vi "tcpServer.vi"(8 "error in (no error)":errorcluster, 11 "TcpServer in":refnum<class "TcpServer.lvclass">) -> (0 "error out":errorcluster, 3 "TcpServer out":refnum<class "TcpServer.lvclass">)   [LabVIEW 2018, in "TcpServer.lvclass"]
doc: "This is the Tcp Server that receives packets from Python Client, send acknowledgement to client and manage the incommiing and outcomming events."
uses:
  TcpServer.lvclass
  TcpServer.lvclass/TcpServer.ctl
panel:
  out "Packet":string
  out "Client IP":string
  out "error tcp":errorcluster
  out "Packet In":string
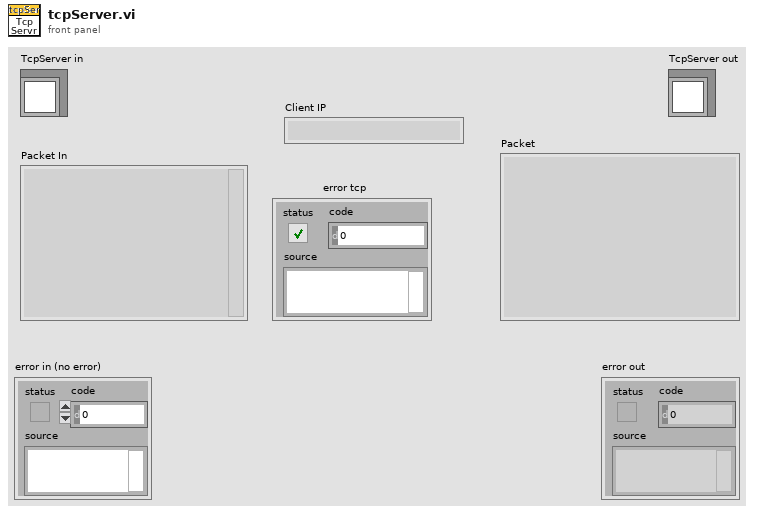
[diagram p1: front panel]
types:
  T1 = typedef "TcpServer.lvclass/userEventsTypeDef.ctl" = cluster{"TcpServer":refnum<user-event>, "Command":refnum<user-event>, "Ack":refnum<user-event>, "Event":refnum<user-event>, "Telemetry":refnum<user-event>}
  T2 = enum16{"Standard", "Buffered", "CRLF", "Immediate"}
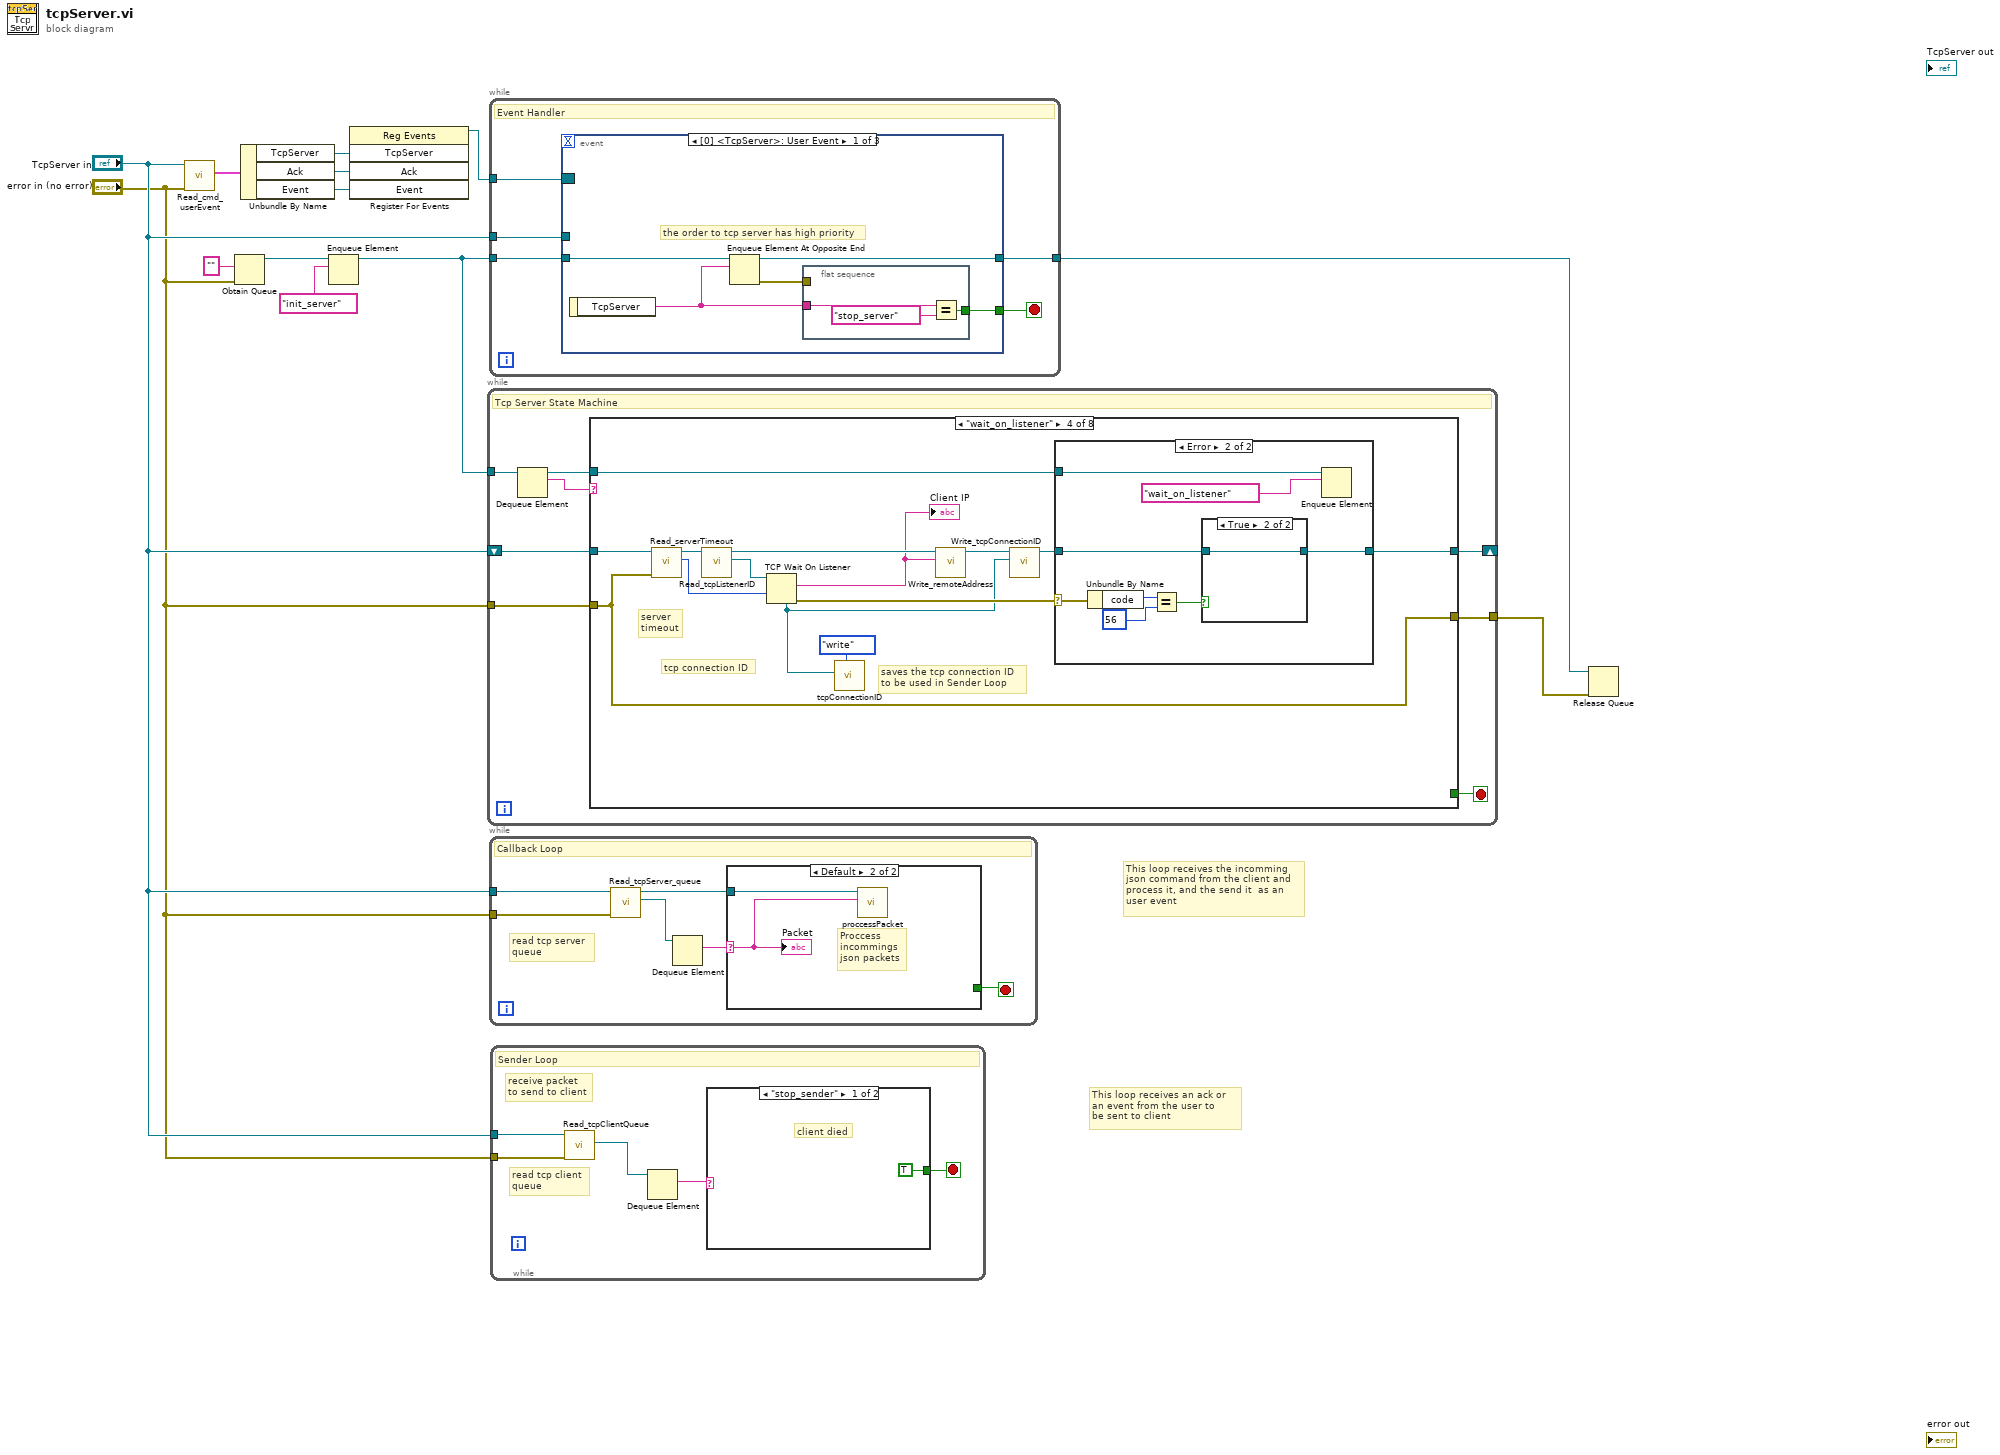
[diagram p0: block diagram]
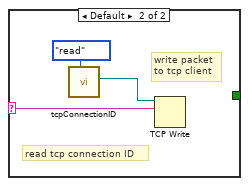
[diagram p2: hidden frame]
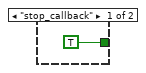
[diagram p3: hidden frame]
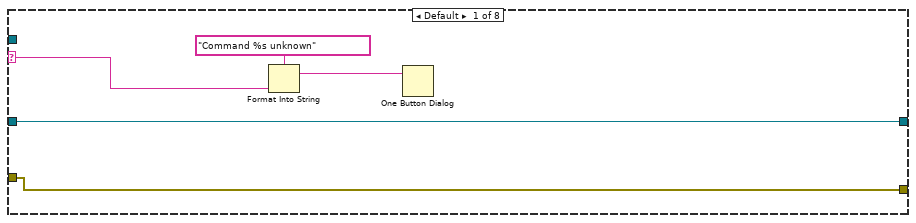
[diagram p4: hidden frame]
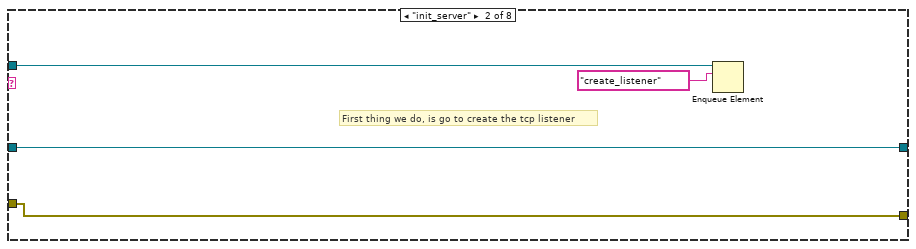
[diagram p5: hidden frame]
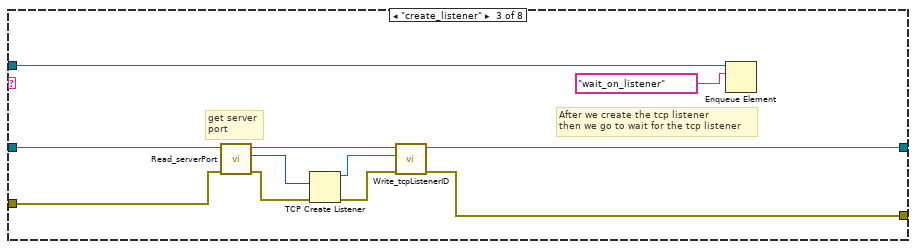
[diagram p6: hidden frame]
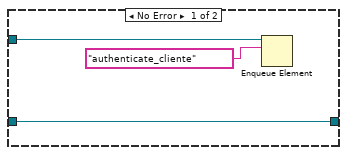
[diagram p7: hidden frame]
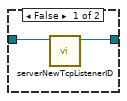
[diagram p8: hidden frame]
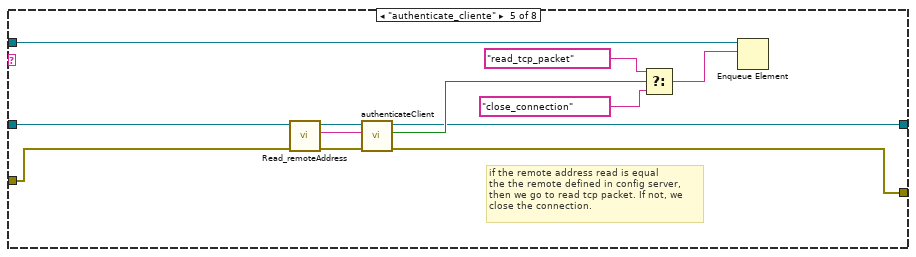
[diagram p9: hidden frame]
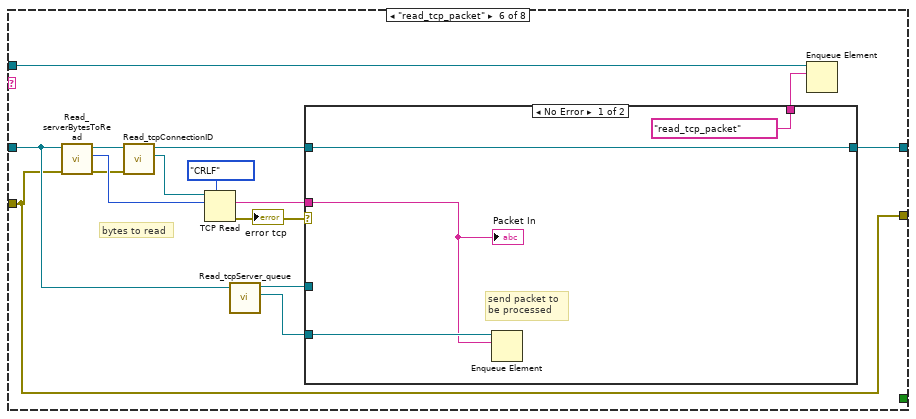
[diagram p10: hidden frame]
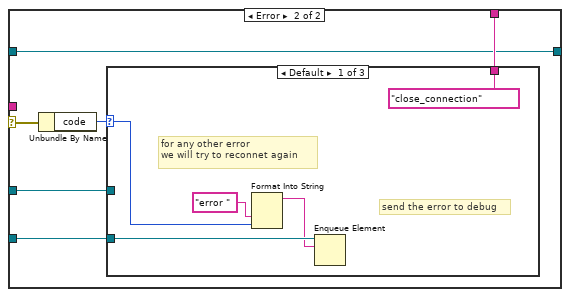
[diagram p11: hidden frame]
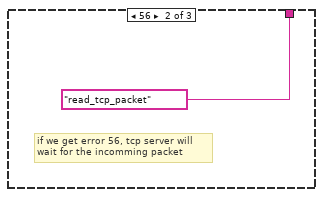
[diagram p12: hidden frame]
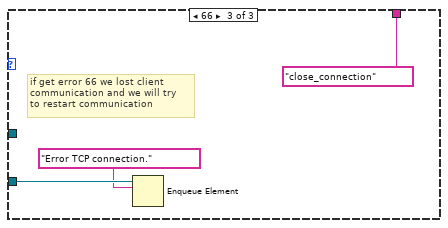
[diagram p13: hidden frame]
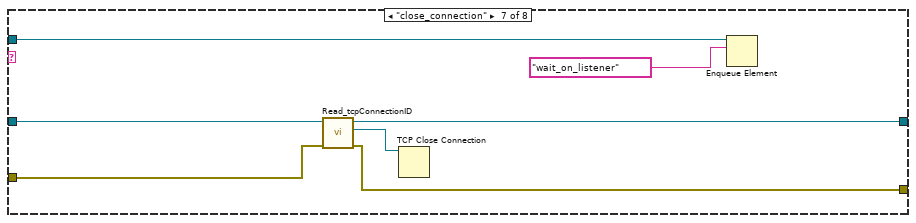
[diagram p14: hidden frame]
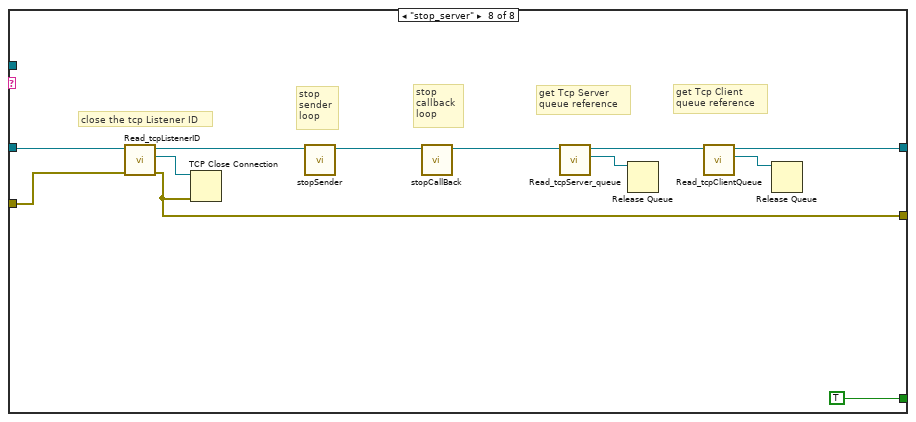
[diagram p15: hidden frame]
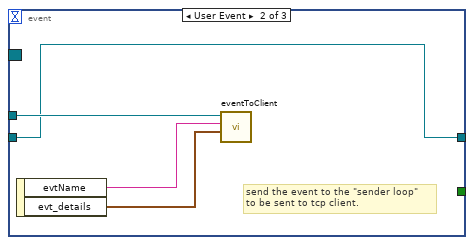
[diagram p16: hidden frame]
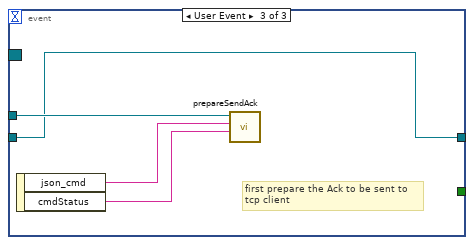
[diagram p17: hidden frame]
diagram:
  # "This loop receives an ack or\nan event from the user to\nbe sent to client"
  # "This loop receives the incomming\njson command from the client and\nprocess it, and the send it  as an \nuser event"
  n1 = call "Read_cmd_userEvent.vi"("error in (no error)"="error in (no error)", "tcpServer in"="TcpServer in") -> ("UserEvents"=w11:T1)  [unwired: 7 in, 2 out]
  n2 = Obtain Queue(element data type="", error in (no error)="error in (no error)") -> (queue out=w12:refnum<queue>)  [unwired: 3 in, 2 out]
  n3 = Unbundle By Name(w11) -> ("TcpServer"=w10:refnum<user-event>, "Ack"=w5:refnum<user-event>, "Event"=w4:refnum<user-event>)
  n4 = Enqueue Element(queue=w12, element="init_server") -> (queue out=w8:refnum<queue>)  [unwired: 2 in, 2 out]
  n5 = register-events(w10, w5, w4) -> (reference out=w9:refnum<event-registration>)  [unwired: 2 in, 1 out]
  n6 = while {
    tunnel: w8 -> [w21]
    shift-right: [w19] -> _
    shift-left: "TcpServer in" -> [w20]
    tunnel: "error in (no error)" -> [w15]
    tunnel: [w14] -> w2
    stop <- w16 stop-if-true
    # "Tcp Server State Machine"
    n7 = Dequeue Element(queue=w21) -> (queue out=w18:refnum<queue>, element=w17:string)  [unwired: 2 in, 2 out]
    n8 = case shown="\"wait_on_listener\"" w17 {
      selector: w17 -> [w25 _ _ _ _ _ _ _]
      tunnel: w20 -> [w23 w30 w39 w52 w81 w90 w122 w133]
      tunnel: [w23 w30 w35 w50 w77 w85 w119 w128] -> w19
      tunnel: w18 -> [_ w29 w34 w49 w76 w88 w121 _]
      tunnel: [_ _ _ _ _ _ _ TRUE] -> w16
      tunnel: w15 -> [w22 w27 w32 w42 w72 w82 w117 w124]
      tunnel: [w22 w27 w31 w42 w70 w82 w116 w123] -> w14
      frame Default {
        n9 = Format Into String(format string="Command %s unknown", w25) -> (resulting string=w24:string)  [unwired: 2 in, 1 out]
        n10 = One Button Dialog(message=w24) -> ()  [unwired: 1 in, 1 out]
      }
      frame "init_server" {
        # "First thing we do, is go to create the tcp listener"
        n11 = Enqueue Element(queue=w29, element="create_listener") -> ()  [unwired: 2 in, 3 out]
      }
      frame "create_listener" {
        # "After we create the tcp listener\nthen we go to wait for the tcp listener"
        # "get server\nport"
        n12 = call "Read_serverPort.vi"("error in (no error)"=w32, "tcpServer in"=w39) -> ("error out"=w40:errorcluster, "serverPort"=w41:u16, "tcpServer out"=w38:refnum<class "TcpServer.lvclass">)  [unwired: 7 in]
        n13 = TCP Create Listener(8:w40, 10:w41) -> (0:w36:errorcluster, 3:w37:refnum<k5>)  [unwired: 3 in, 1 out]
        n14 = call "Write_tcpListenerID.vi"("error in (no error)"=w36, "tcpListenerID"=w37, "tcpServer in"=w38) -> ("error out"=w31:errorcluster, "tcpServer out"=w35:refnum<class "TcpServer.lvclass">)  [unwired: 7 in]
        n15 = Enqueue Element(queue=w34, element="wait_on_listener") -> ()  [unwired: 2 in, 3 out]
      }
      frame "wait_on_listener" {
        # "tcp connection ID"
        # "saves the tcp connection ID\nto be used in Sender Loop"
        # "server\ntimeout"
        n16 = call "Read_serverTimeout.vi"("error in (no error)"=w42, "tcpServer in"=w52) -> ("serverTimeout"=w53:i32, "tcpServer out"=w54:refnum<class "TcpServer.lvclass">)  [unwired: 7 in, 1 out]
        n17 = call "Read_tcpListenerID.vi"("tcpServer in"=w54) -> ("tcpListenerID"=w55:refnum<k5>, "tcpServer out"=w48:refnum<class "TcpServer.lvclass">)  [unwired: 8 in, 1 out]
        n18 = TCP Wait On Listener(9:w53, 11:w55) -> (0:w51:errorcluster, 2:w45:string, 4:w43:refnum<k5>)  [unwired: 2 in, 2 out]
        "Client IP" <- w45
        n19 = call "tcpConnectionID.vi"("function"=enum16{"read", "write"}."write", "connection ID"=w43) -> ()  [unwired: 9 in, 1 out]
        n20 = call "Write_remoteAddress.vi"("remoteAddress"=w45, "TcpServer in"=w48) -> ("TcpServer out"=w46:refnum<class "TcpServer.lvclass">)  [unwired: 8 in, 1 out]
        n21 = call "Write_tcpConnectionID.vi"("tcpConnectionID"=w43, "TcpServer in"=w46) -> ("TcpServer out"=w47:refnum<class "TcpServer.lvclass">)  [unwired: 8 in, 1 out]
        n22 = case shown="Error" w51 {
          selector: w51 -> [_ w64]
          tunnel: w47 -> [w58 w62]
          tunnel: [w58 w61] -> w50
          tunnel: w49 -> [w56 w60]
          frame No Error {
            n23 = Enqueue Element(queue=w56, element="authenticate_cliente") -> ()  [unwired: 2 in, 3 out]
          }
          frame Error {
            n24 = Unbundle By Name(w64) -> ("code"=w66:i32)
            n25 = Equal?(x=w66, y=56) -> (x = y?=w63:bool)
            n26 = case shown="True" w63 {
              tunnel: w62 -> [w68 w69]
              tunnel: [w67 w69] -> w61
              frame False {
                n27 = call "serverNewTcpListenerID.vi"("tcpServer in"=w68) -> ("tcpServer out"=w67:refnum<class "TcpServer.lvclass">)  [unwired: 9 in, 1 out]
              }
              frame True {
              }
            }
            n28 = Enqueue Element(queue=w60, element="wait_on_listener") -> ()  [unwired: 2 in, 3 out]
          }
        }
      }
      frame "authenticate_cliente" {
        # "if the remote address read is equal\nthe the remote defined in config server,\nthen we go to read tcp packet. If not, we\nclose the connection."
        n29 = call "Read_remoteAddress.vi"("error in (no error)"=w72, "TcpServer in"=w81) -> ("error out"=w71:errorcluster, "remoteAddress"=w73:string, "TcpServer out"=w74:refnum<class "TcpServer.lvclass">)  [unwired: 7 in]
        n30 = call "authenticateClient.vi"("error in (no error)"=w71, "Computer Name"=w73, "tcpServer in"=w74) -> ("error out"=w70:errorcluster, "authenticate"=w80:bool, "tcpServer out"=w77:refnum<class "TcpServer.lvclass">)  [unwired: 6 in]
        n31 = Select(t="read_tcp_packet", s=w80, f="close_connection") -> (s? t:f=w75:string)
        n32 = Enqueue Element(queue=w76, element=w75) -> ()  [unwired: 2 in, 3 out]
      }
      frame "read_tcp_packet" {
        # "bytes to read"
        n33 = call "Read_serverBytesToRead.vi"("error in (no error)"=w82, "tcpServer in"=w90) -> ("error out"=w83:errorcluster, "serverBytesToRead"=w93:i32, "tcpServer out"=w89:refnum<class "TcpServer.lvclass">)  [unwired: 7 in]
        n34 = call "Read_tcpConnectionID.vi"("error in (no error)"=w83, "TcpServer in"=w89) -> ("tcpConnectionID"=w84:refnum<k5>, "TcpServer out"=w86:refnum<class "TcpServer.lvclass">)  [unwired: 7 in, 1 out]
        n35 = TCP Read(connection ID=w84, bytes to read=w93, 7:T2."CRLF" ("mode (standard)")) -> (data out=w96:string, error out=w94:errorcluster)  [unwired: 2 in, 1 out]
        "error tcp" <- w94
        n36 = call "Read_tcpServer_queue.vi"("tcpServer in"=w90) -> ("tcpServer queue"=w92:refnum<queue>, "tcpServer out"=w91:refnum<class "TcpServer.lvclass">)  [unwired: 8 in, 1 out]
        n37 = case shown="No Error" w94 {
          selector: w94 -> [_ w106]
          tunnel: w96 -> [w97 _]
          tunnel: w92 -> [w100 w104]
          tunnel: w91 -> [_ w103]
          tunnel: ["read_tcp_packet" w102] -> w87
          tunnel: w86 -> [w98 w101]
          tunnel: [w98 w101] -> w85
          frame No Error {
            # "send packet to\nbe processed"
            n38 = Enqueue Element(queue=w100, element=w97) -> ()  [unwired: 2 in, 3 out]
            "Packet In" <- w97
          }
          frame Error {
            n39 = Unbundle By Name(w106) -> ("code"=w105:i32)
            n40 = case shown="Default" w105 {
              selector: w105 -> [w110 _ _]
              tunnel: w104 -> [w109 _ w115]
              tunnel: w103 -> [_ _ _]
              tunnel: ["close_connection" "read_tcp_packet" "close_connection"] -> w102
              frame Default {
                # "send the error to debug"
                # "for any other error\nwe will try to reconnet again"
                n41 = Format Into String("error ", w110) -> (resulting string=w108:string)  [unwired: 3 in, 1 out]
                n42 = Enqueue Element(queue=w109, element=w108) -> ()  [unwired: 2 in, 3 out]
              }
              frame 56 {
                # "if we get error 56, tcp server will \nwait for the incomming packet"
              }
              frame 66 {
                # "if get error 66 we lost client \ncommunication and we will try\nto restart communication"
                n43 = Enqueue Element(queue=w115, element="Error TCP connection.") -> ()  [unwired: 2 in, 3 out]
              }
            }
          }
        }
        n44 = Enqueue Element(queue=w88, element=w87) -> ()  [unwired: 2 in, 3 out]
      }
      frame "close_connection" {
        n45 = call "Read_tcpConnectionID.vi"("error in (no error)"=w117, "TcpServer in"=w122) -> ("error out"=w116:errorcluster, "tcpConnectionID"=w118:refnum<k5>, "TcpServer out"=w119:refnum<class "TcpServer.lvclass">)  [unwired: 7 in]
        n46 = TCP Close Connection(connection ID=w118) -> ()  [unwired: 2 in, 2 out]
        n47 = Enqueue Element(queue=w121, element="wait_on_listener") -> ()  [unwired: 2 in, 3 out]
      }
      frame "stop_server" {
        # "close the tcp Listener ID"
        # "stop\nsender\nloop"
        # "stop\ncallback\nloop"
        # "get Tcp Client \nqueue reference"
        # "get Tcp Server \nqueue reference"
        n48 = call "Read_tcpListenerID.vi"("error in (no error)"=w124, "tcpServer in"=w133) -> ("error out"=w123:errorcluster, "tcpListenerID"=w134:refnum<k5>, "tcpServer out"=w126:refnum<class "TcpServer.lvclass">)  [unwired: 7 in]
        n49 = TCP Close Connection(connection ID=w134, error in (no error)=w123) -> ()  [unwired: 1 in, 2 out]
        n50 = call "stopSender.vi"("TcpServer in"=w126) -> ("TcpServer out"=w127:refnum<class "TcpServer.lvclass">)  [unwired: 9 in, 1 out]
        n51 = call "stopCallBack.vi"("TcpServer in"=w127) -> ("TcpServer out"=w125:refnum<class "TcpServer.lvclass">)  [unwired: 9 in, 1 out]
        n52 = call "Read_tcpServer_queue.vi"("tcpServer in"=w125) -> ("tcpServer queue"=w131:refnum<queue>, "tcpServer out"=w130:refnum<class "TcpServer.lvclass">)  [unwired: 8 in, 1 out]
        n53 = Release Queue(queue=w131) -> ()  [unwired: 2 in, 3 out]
        n54 = call "Read_tcpClientQueue.vi"("tcpServer in"=w130) -> ("tcpClient queue"=w129:refnum<queue>, "tcpServer out"=w128:refnum<class "TcpServer.lvclass">)  [unwired: 8 in, 1 out]
        n55 = Release Queue(queue=w129) -> ()  [unwired: 2 in, 3 out]
      }
    }
  }
  n56 = while {
    tunnel: w8 -> [w139]
    tunnel: w9 -> [w138]
    tunnel: [w136] -> w6
    tunnel: "TcpServer in" -> [w135]
    stop <- w137 stop-if-true
    # "Event Handler"
    n57 = event shown="[0] <TcpServer>: User Event" {
      selector: w138 -> [_ _ _]
      dyn-events: _ -> [_ _ _]
      timeout: _ -> [_ _ _]
      tunnel: w139 -> [w144 w148 w152]
      tunnel: [w142 _ _] -> w137
      tunnel: [w140 w148 w152] -> w136
      tunnel: w135 -> [_ w151 w155]
      event User Event {
        # "the order to tcp server has high priority"
        n58 = event-data() -> ("TcpServer"=w143:string)  [unwired: 1 in]
        n59 = Enqueue Element At Opposite End(queue=w144, element=w143) -> (queue out=w140:refnum<queue>, error out=w141:errorcluster)  [unwired: 2 in, 1 out]
        n60 = flat-sequence {
          tunnel: w143 -> [w147]
          tunnel: [w145] -> w142
          tunnel: w141 -> [_]
          frame #0 {
            n61 = Equal?(x=w147, y="stop_server") -> (x = y?=w145:bool)
          }
        }
      }
      event User Event {
        # "send the event to the \"sender loop\"\nto be sent to tcp client."
        n62 = event-data() -> ("evtName"=w150:string, "evt_details"=w149:cluster{"state":i32})  [unwired: 1 in]
        n63 = call "eventToClient.vi"("evt_details"=w149, "evtName"=w150, "TcpServer in"=w151) -> ()  [unwired: 7 in, 2 out]
      }
      event User Event {
        # "first prepare the Ack to be sent to\ntcp client"
        n64 = event-data() -> ("json_cmd"=w154:string, "cmdStatus"=w153:string)  [unwired: 1 in]
        n65 = call "prepareSendAck.vi"("cmdStatus"=w153, "Ack"=w154, "tcpServer in"=w155) -> ()  [unwired: 7 in, 2 out]
      }
    }
  }
  n66 = while {
    tunnel: "TcpServer in" -> [w157]
    tunnel: "error in (no error)" -> [w156]
    stop <- w158 stop-if-true
    # "read tcp server \nqueue"
    # "Callback Loop"
    n67 = call "Read_tcpServer_queue.vi"("error in (no error)"=w156, "tcpServer in"=w157) -> ("tcpServer queue"=w161:refnum<queue>, "tcpServer out"=w160:refnum<class "TcpServer.lvclass">)  [unwired: 7 in, 1 out]
    n68 = Dequeue Element(queue=w161) -> (element=w159:string)  [unwired: 2 in, 3 out]
    n69 = case shown="Default" w159 {
      selector: w159 -> [_ w163]
      tunnel: w160 -> [_ w164]
      tunnel: [TRUE _] -> w158
      frame "stop_callback" {
      }
      frame Default {
        # "Proccess\nincommings\njson packets"
        n70 = call "proccessPacket.vi"("tcp packet"=w163, "tcpServer in"=w164) -> ()  [unwired: 8 in, 2 out]
        "Packet" <- w163
      }
    }
  }
  n71 = while {
    tunnel: "TcpServer in" -> [w169]
    tunnel: "error in (no error)" -> [w165]
    stop <- w167 stop-if-true
    # "receive packet\nto send to client"
    # "read tcp client \nqueue"
    # "Sender Loop"
    n72 = call "Read_tcpClientQueue.vi"("error in (no error)"=w165, "tcpServer in"=w169) -> ("tcpClient queue"=w166:refnum<queue>)  [unwired: 7 in, 2 out]
    n73 = Dequeue Element(queue=w166) -> (element=w168:string)  [unwired: 2 in, 3 out]
    n74 = case shown="\"stop_sender\"" w168 {
      selector: w168 -> [_ w173]
      tunnel: [TRUE _] -> w167
      frame "stop_sender" {
        # "client died"
      }
      frame Default {
        # "write packet\nto tcp client"
        # "read tcp connection ID"
        n75 = call "tcpConnectionID.vi"("function"=enum16{"read", "write"}."read") -> ("connection ID out"=w171:refnum<k5>)  [unwired: 10 in]
        n76 = TCP Write(connection ID=w171, data in=w173) -> ()  [unwired: 2 in, 3 out]
      }
    }
  }
  n77 = Release Queue(queue=w6, error in (no error)=w2) -> ()  [unwired: 1 in, 3 out]
